vi "Retain Overflow Bits (SubVI).vi"(7 "N Overflow Bits":u8, 8 "Bit Array In":bool[](array[boolean])=[FALSE, FALSE, FALSE, FALSE, FALSE, FALSE, FALSE, FALSE], 11 "Bit Depth":u8) -> (3 "Bit Array Out":bool[](array[boolean]))   [LabVIEW 2014]
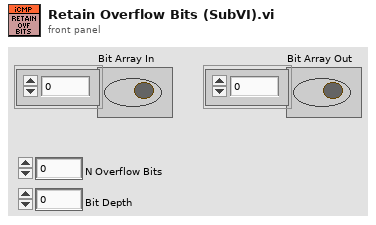
[diagram p1: front panel]
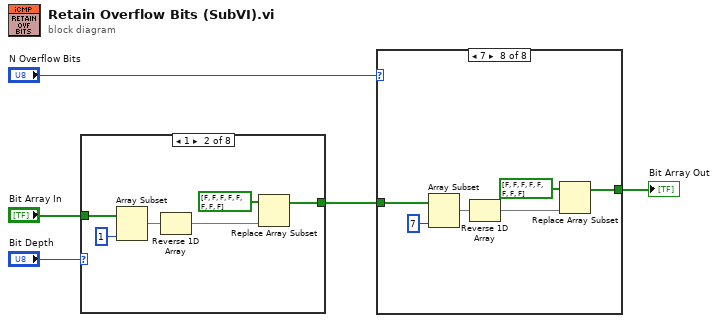
[diagram p0: block diagram]
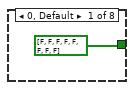
[diagram p2: hidden frame]
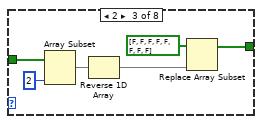
[diagram p3: hidden frame]
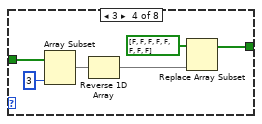
[diagram p4: hidden frame]
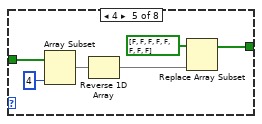
[diagram p5: hidden frame]
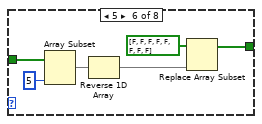
[diagram p6: hidden frame]
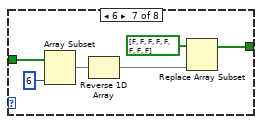
[diagram p7: hidden frame]
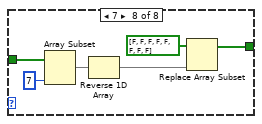
[diagram p8: hidden frame]
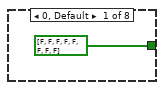
[diagram p9: hidden frame]
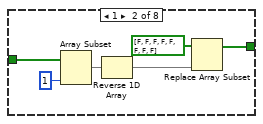
[diagram p10: hidden frame]
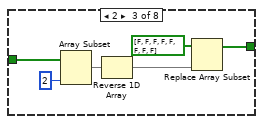
[diagram p11: hidden frame]
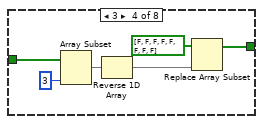
[diagram p12: hidden frame]
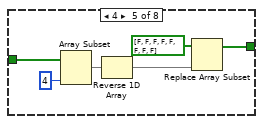
[diagram p13: hidden frame]
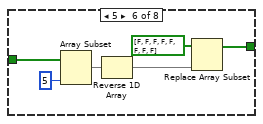
[diagram p14: hidden frame]
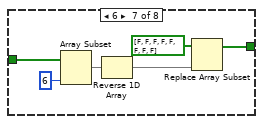
[diagram p15: hidden frame]
diagram:
  n1 = case shown="1" "Bit Depth" {
    tunnel: [bool[] [FALSE, FALSE, FALSE, FALSE, FALSE, FALSE, FALSE, FALSE] w8 w14 w20 w26 w32 w38 w44] -> w3
    tunnel: "Bit Array In" -> [_ w11 w17 w23 w29 w35 w41 w47]
    frame 0, Default {
    }
    frame 1 {
      n2 = Array Subset(array=w11, length=1) -> (w12:bool[])  [unwired: 1 in]
      n3 = Reverse 1D Array(array=w12) -> (reversed array=w9:bool[])
      n4 = Replace Array Subset(array=bool[] [FALSE, FALSE, FALSE, FALSE, FALSE, FALSE, FALSE, FALSE], new element=w9) -> (w8:bool[])  [unwired: 1 in]
    }
    frame 2 {
      n5 = Array Subset(array=w17, length=2) -> (w18:bool[])  [unwired: 1 in]
      n6 = Reverse 1D Array(array=w18) -> (reversed array=w15:bool[])
      n7 = Replace Array Subset(array=bool[] [FALSE, FALSE, FALSE, FALSE, FALSE, FALSE, FALSE, FALSE], new element=w15) -> (w14:bool[])  [unwired: 1 in]
    }
    frame 3 {
      n8 = Array Subset(array=w23, length=3) -> (w24:bool[])  [unwired: 1 in]
      n9 = Reverse 1D Array(array=w24) -> (reversed array=w21:bool[])
      n10 = Replace Array Subset(array=bool[] [FALSE, FALSE, FALSE, FALSE, FALSE, FALSE, FALSE, FALSE], new element=w21) -> (w20:bool[])  [unwired: 1 in]
    }
    frame 4 {
      n11 = Array Subset(array=w29, length=4) -> (w30:bool[])  [unwired: 1 in]
      n12 = Reverse 1D Array(array=w30) -> (reversed array=w27:bool[])
      n13 = Replace Array Subset(array=bool[] [FALSE, FALSE, FALSE, FALSE, FALSE, FALSE, FALSE, FALSE], new element=w27) -> (w26:bool[])  [unwired: 1 in]
    }
    frame 5 {
      n14 = Array Subset(array=w35, length=5) -> (w36:bool[])  [unwired: 1 in]
      n15 = Reverse 1D Array(array=w36) -> (reversed array=w33:bool[])
      n16 = Replace Array Subset(array=bool[] [FALSE, FALSE, FALSE, FALSE, FALSE, FALSE, FALSE, FALSE], new element=w33) -> (w32:bool[])  [unwired: 1 in]
    }
    frame 6 {
      n17 = Array Subset(array=w41, length=6) -> (w42:bool[])  [unwired: 1 in]
      n18 = Reverse 1D Array(array=w42) -> (reversed array=w39:bool[])
      n19 = Replace Array Subset(array=bool[] [FALSE, FALSE, FALSE, FALSE, FALSE, FALSE, FALSE, FALSE], new element=w39) -> (w38:bool[])  [unwired: 1 in]
    }
    frame 7 {
      n20 = Array Subset(array=w47, length=7) -> (w48:bool[])  [unwired: 1 in]
      n21 = Reverse 1D Array(array=w48) -> (reversed array=w45:bool[])
      n22 = Replace Array Subset(array=bool[] [FALSE, FALSE, FALSE, FALSE, FALSE, FALSE, FALSE, FALSE], new element=w45) -> (w44:bool[])  [unwired: 1 in]
    }
  }
  n23 = case shown="7" "N Overflow Bits" {
    tunnel: w3 -> [_ w55 w61 w67 w73 w79 w85 w91]
    tunnel: [bool[] [FALSE, FALSE, FALSE, FALSE, FALSE, FALSE, FALSE, FALSE] w50 w56 w62 w68 w74 w80 w86] -> w5
    frame 0, Default {
    }
    frame 1 {
      n24 = Array Subset(array=w55, length=1) -> (w54:bool[])  [unwired: 1 in]
      n25 = Reverse 1D Array(array=w54) -> (reversed array=w53:bool[])
      n26 = Replace Array Subset(array=bool[] [FALSE, FALSE, FALSE, FALSE, FALSE, FALSE, FALSE, FALSE], new element=w53) -> (w50:bool[])  [unwired: 1 in]
    }
    frame 2 {
      n27 = Array Subset(array=w61, length=2) -> (w60:bool[])  [unwired: 1 in]
      n28 = Reverse 1D Array(array=w60) -> (reversed array=w59:bool[])
      n29 = Replace Array Subset(array=bool[] [FALSE, FALSE, FALSE, FALSE, FALSE, FALSE, FALSE, FALSE], new element=w59) -> (w56:bool[])  [unwired: 1 in]
    }
    frame 3 {
      n30 = Array Subset(array=w67, length=3) -> (w66:bool[])  [unwired: 1 in]
      n31 = Reverse 1D Array(array=w66) -> (reversed array=w65:bool[])
      n32 = Replace Array Subset(array=bool[] [FALSE, FALSE, FALSE, FALSE, FALSE, FALSE, FALSE, FALSE], new element=w65) -> (w62:bool[])  [unwired: 1 in]
    }
    frame 4 {
      n33 = Array Subset(array=w73, length=4) -> (w72:bool[])  [unwired: 1 in]
      n34 = Reverse 1D Array(array=w72) -> (reversed array=w71:bool[])
      n35 = Replace Array Subset(array=bool[] [FALSE, FALSE, FALSE, FALSE, FALSE, FALSE, FALSE, FALSE], new element=w71) -> (w68:bool[])  [unwired: 1 in]
    }
    frame 5 {
      n36 = Array Subset(array=w79, length=5) -> (w78:bool[])  [unwired: 1 in]
      n37 = Reverse 1D Array(array=w78) -> (reversed array=w77:bool[])
      n38 = Replace Array Subset(array=bool[] [FALSE, FALSE, FALSE, FALSE, FALSE, FALSE, FALSE, FALSE], new element=w77) -> (w74:bool[])  [unwired: 1 in]
    }
    frame 6 {
      n39 = Array Subset(array=w85, length=6) -> (w84:bool[])  [unwired: 1 in]
      n40 = Reverse 1D Array(array=w84) -> (reversed array=w83:bool[])
      n41 = Replace Array Subset(array=bool[] [FALSE, FALSE, FALSE, FALSE, FALSE, FALSE, FALSE, FALSE], new element=w83) -> (w80:bool[])  [unwired: 1 in]
    }
    frame 7 {
      n42 = Array Subset(array=w91, length=7) -> (w90:bool[])  [unwired: 1 in]
      n43 = Reverse 1D Array(array=w90) -> (reversed array=w89:bool[])
      n44 = Replace Array Subset(array=bool[] [FALSE, FALSE, FALSE, FALSE, FALSE, FALSE, FALSE, FALSE], new element=w89) -> (w86:bool[])  [unwired: 1 in]
    }
  }
  "Bit Array Out" <- w5
